vi "add_counter_data.vi"(8 "error in (no error)":errorcluster, 10 "counter data":string[](array[string]), 11 "Analysis in":refnum<class "Analysis.lvclass">) -> (0 "error out":errorcluster, 3 "Analysis out":refnum<class "Analysis.lvclass">)   [LabVIEW 2018, in "Analysis.lvclass"]
doc: "adds the data to the CounterArray\nswitch_name, counter"
uses:
  Analysis.lvclass
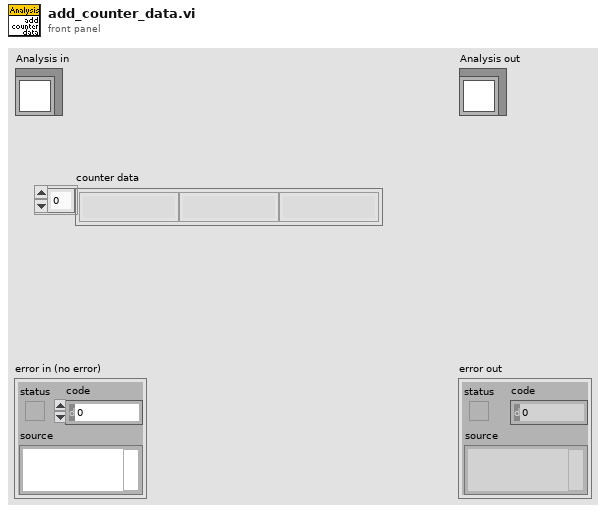
[diagram p1: front panel]
types:
  T1 = typedef "CounterArray.ctl" = string[][]
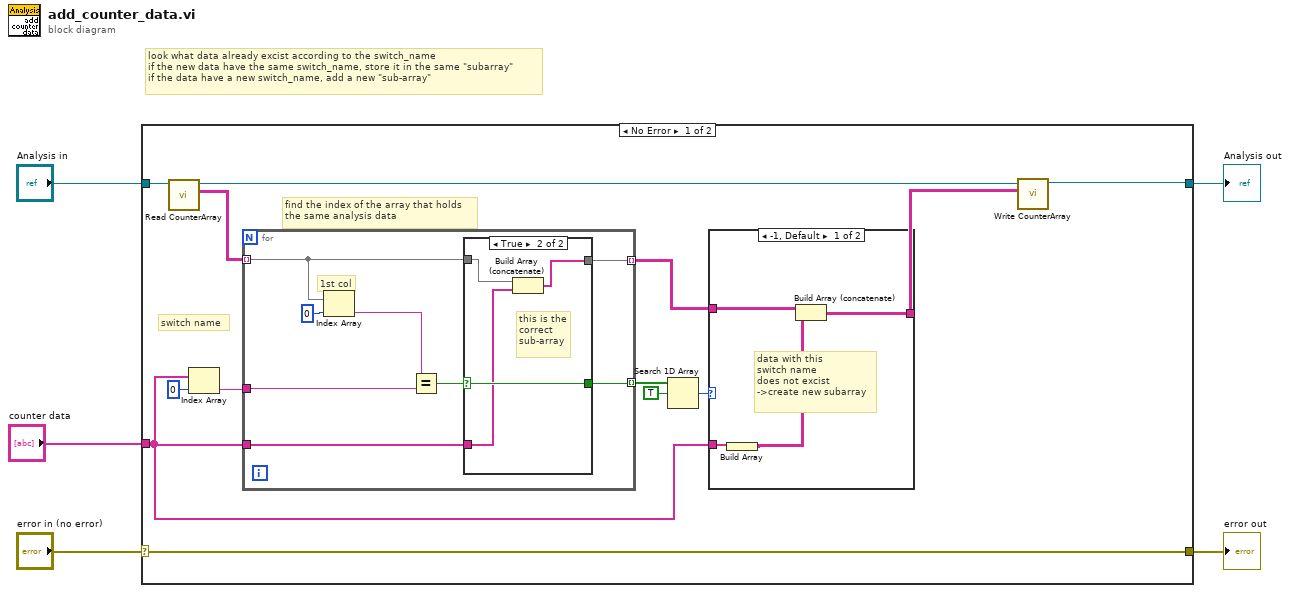
[diagram p0: block diagram]
diagram:
  # "look what data already excist according to the switch_name\nif the new data have the same switch_name, store it in the same \"subarray\"\nif the data have a new switch_name, add a new \"sub-array\""
  n1 = case shown="No Error" "error in (no error)" {
    selector: "error in (no error)" -> [w18 w39]
    tunnel: [w18 w39] -> w4
    tunnel: [w15 w38] -> w2
    tunnel: "Analysis in" -> [w17 w38]
    tunnel: "counter data" -> [w7 _]
    frame No Error {
      # "find the index of the array that holds\nthe same analysis data"
      # "switch name"
      n2 = call-dynamic "Read CounterArray.vi"("Analysis in"=w17) -> ("CounterArray"=w8:T1, "Analysis out"=w16:refnum<class "Analysis.lvclass">)  [unwired: 8 in, 1 out]
      n3 = Index Array(array=w7, index=0) -> (element=w12:string)
      n4 = for {
        tunnel: w8 -> [w27] mode=indexing
        tunnel: w12 -> [w31]
        tunnel: [w28] -> w13 mode=indexing
        tunnel: [w26] -> w9 mode=indexing
        tunnel: w7 -> [w30]
        # "1st col"
        n5 = Index Array(array=w27, index=0 ("disabled index (col)")) -> (element=w24:string)
        n6 = Equal?(x=w24, y=w31) -> (x = y?=w29:bool)
        n7 = case shown="True" w29 {
          selector: w29 -> [w33 w37]
          tunnel: w30 -> [_ w34]
          tunnel: [w33 w37] -> w28
          tunnel: w27 -> [w32 w36]
          tunnel: [w32 w35] -> w26
          frame False {
            # "not the right\nsub-array"
          }
          frame True {
            # "this is the\ncorrect\nsub-array"
            n8 = Build Array (concatenate)(w36, w34) -> (w35:string[])
          }
        }
      }
      n9 = Search 1D Array(1D array=w13, element=TRUE) -> (index of element=w10:i32)  [unwired: 1 in]
      n10 = case shown="-1, Default" w10 {
        tunnel: w9 -> [w20 w23]
        tunnel: w7 -> [w22 _]
        tunnel: [w21 w23] -> w6
        frame -1, Default {
          # "data with this\nswitch name\ndoes not excist\n->create new subarray"
          n11 = Build Array(w22) -> (w19:string[][])
          n12 = Build Array (concatenate)(w20, w19) -> (w21:string[][])
        }
        frame 0.. {
          # "all fine, data have been\ninserted already"
        }
      }
      n13 = call-dynamic "Write CounterArray.vi"("CounterArray"=w6, "Analysis in"=w16) -> ("Analysis out"=w15:refnum<class "Analysis.lvclass">)  [unwired: 8 in, 1 out]
    }
    frame Error {
    }
  }
  "error out" <- w4
  "Analysis out" <- w2
